vi "subvi_Save_tdms.vi"(6 "data":waveform(dbl)[](array[waveform]), 7 "그룹 이름":string, 8 "Error In":errorcluster caption="에러 입력", 9 "Save name":string="FileNAME", 11 "appended path":path) -> (0 "Error Out":errorcluster caption="에러 출력")   [LabVIEW 2016]
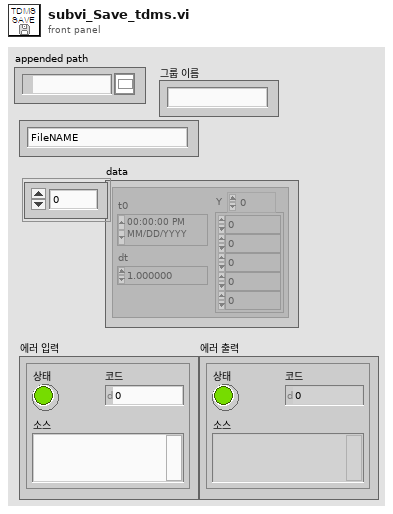
[diagram p1: front panel]
types:
  T1 = enum16{"open", "open or create", "create or replace", "create", "open (read-only)"}
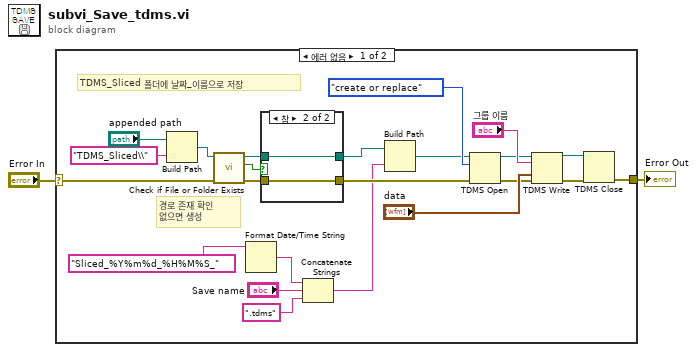
[diagram p0: block diagram]
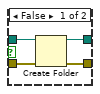
[diagram p2: hidden frame]
diagram:
  n1 = case shown="에러 없음" "Error In" {
    selector: "Error In" -> [w14 w32]
    tunnel: [w18 w32] -> w1
    frame No Error {
      # "TDMS_Sliced 폴더에 날짜_이름으로 저장"
      # "경로 존재 확인\n없으면 생성"
      n2 = Build Path(base path="appended path", name or relative path="TDMS_Sliced\\" ("문자열")) -> (appended path=w10:path)
      n3 = call <vilib>:"Check if File or Folder Exists.vi"("error in (no error)"=w14, "path"=w10) -> ("error out"=w15:errorcluster, "file or folder exists?"=w17:bool, "dup path"=w16:path)  [unwired: 7 in]
      n4 = Format Date/Time String(time format string (%c)="Sliced_%Y%m%d_%H%M%S_" ("시간 포맷 문자열 (%c)")) -> (date/time string=w8:string)  [unwired: 2 in]
      n5 = case shown="참" w17 {
        tunnel: w16 -> [w29 w31]
        tunnel: w15 -> [w28 w30]
        tunnel: [w26 w31] -> w3
        tunnel: [w27 w30] -> w13
        frame False {
          n6 = Create Folder(path (use dialog)=w29, error in=w28) -> (created path=w26:path, error out=w27:errorcluster)  [unwired: 1 in, 1 out]
        }
        frame True {
        }
      }
      n7 = Concatenate Strings(w8, "Save name", ".tdms" ("문자열")) -> (w9:string)
      n8 = Build Path(base path=w3, name or relative path=w9) -> (appended path=w4:path)
      n9 = TDMS Open(8:w13, 10:T1."create or replace" ("동작(0:open)"), 11:w4) -> (0:w20:errorcluster, 3:w21:refnum<k34>)  [unwired: 4 in]
      n10 = TDMS Write(0:w21, 5:"그룹 이름", 9:"data", 11:w20) -> (4:w22:refnum<k34>, 15:w19:errorcluster)  [unwired: 2 in, 2 out]
      n11 = TDMS Close(8:w19, 11:w22) -> (0:w18:errorcluster)  [unwired: 1 out]
    }
    frame Error {
    }
  }
  "Error Out" <- w1
